vi "Read Pots.vi"() -> (2 "Right Pot":dbl, 3 "Left Pot":dbl, 4 "Right Unzeroed":dbl, 6 "Left Unzeroed":dbl)   [LabVIEW 2014]
uses:
  Robot Global Data.vi
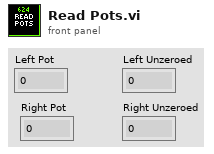
[diagram p1: front panel]
types:
  T1 = typedef "Dashboard Control Data.ctl" = cluster{"Cam Exposure":dbl, "Go to angle":dbl, "Steer PID Gains":cluster{"proportional gain (Kc)":dbl, "integral time (Ti, min)":dbl, "derivative time (Td, min)":dbl}, "Steer PID output Range":cluster{"output high":dbl, "output low":dbl}, "Pressure m \nValue":dbl, "Pressure b \nValue":dbl, "Strafe Timer\nWait":dbl, "Roller Command Cluster ":T2, "Elevator":T3, "Strafe Correct min X":dbl, "IMU Enable":bool, "Encoder Control":T5}
  T2 = typedef "Roller Control.ctl" = cluster{"Left Roller Speed":dbl, "Right Roller Speed":dbl, "Left Roller Speed Back":dbl, "Right Roller Speed Back":dbl, "Roller Align Decide Limit":u32, "Left Roller Speed Unload":dbl, "Right Roller Speed Unload":dbl, "Ping Dist Difference":dbl, "Ping In Dist":dbl, "Right Pot 0":dbl, "Pot Threshold":dbl, "Left Pot 0":dbl, "Manual 0s?":bool, "Right Pot Scale":dbl, "Left Pot Scale":dbl, "0 wait time":i32, "Reset?":bool}
  T3 = typedef "Elevator DB Control.ctl" = cluster{"PID Output Range":cluster{"output high":dbl, "output low":dbl}, "PID gains":cluster{"proportional gain (Kc)":dbl, "integral time (Ti, min)":dbl, "derivative time (Td, min)":dbl}, "Height Tolerance":dbl, " Encoder Constant":dbl, "Safe Mode Max Speed":dbl, "Eject Time":dbl, "Encoder Filter?":bool, "Zeroing Speed":dbl, "Presets":T4}
  T4 = typedef "Elevator Presets.ctl" = cluster{"Hold Tote":dbl, "Hold Trashcan":dbl, "Pickup 2 w/ Tote":dbl, "Pickup 2 w/ Trashcan":dbl, "Pickup 3 w/ Tote":dbl, "Pickup 3 w/ Trashcan":dbl, "Bottom":dbl, "Pickup 1 w/ Tote":dbl, "Pickup Trashcan":dbl, "Pickup 1 w/ Trashcan":dbl, "Eject":dbl}
  T5 = typedef "Encoder Control.ctl" = cluster{"Left Tick Constant":dbl, "Right Tick Constant":dbl, "Center Tick Constant":dbl, "Reset?":bool}
  T6 = typedef "WPI_PotentiometerDevRef.ctl" = cluster{"DevStatus":errorcluster, "Controller":T7, "Analog Channel":T8, "Invert Output":bool}
  T7 = typedef "FPGA_TypedefAnalogModule.ctl" = enum16{"Controller 1"}
  T8 = typedef "FPGA_AIChannel.ctl" = enum8{"AI 0", "AI 1", "AI 2", "AI 3", "AI MXP 0", "AI MXP 1", "AI MXP 2", "AI MXP 3", "Invalid"}
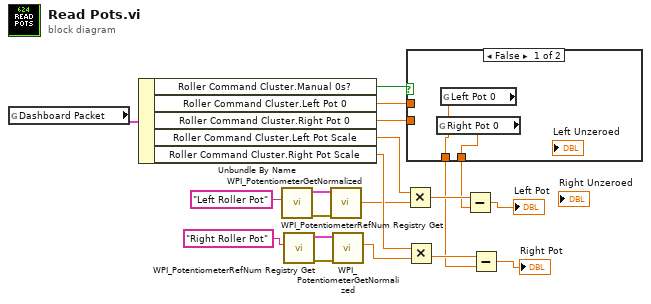
[diagram p0: block diagram]
diagram:
  n1 = global read "Robot Global Data.vi" "Dashboard Packet"() -> (w14:T1)
  n2 = Unbundle By Name(w14) -> ("Roller Command Cluster.Manual 0s?"=w5:bool, "Roller Command Cluster.Left Pot 0"=w4:dbl, "Roller Command Cluster.Right Pot 0"=w2:dbl, "Roller Command Cluster.Left Pot Scale"=w13:dbl, "Roller Command Cluster.Right Pot Scale"=w12:dbl)
  n3 = call <vilib>:"WPI_PotentiometerRefNum Registry Get.vi"("refnum name"="Left Roller Pot") -> ("error out"=w17:errorcluster, "PotDevRef"=w18:T6)  [unwired: 9 in]
  n4 = call <vilib>:"WPI_PotentiometerRefNum Registry Get.vi"("refnum name"="Right Roller Pot") -> ("error out"=w20:errorcluster, "PotDevRef"=w19:T6)  [unwired: 9 in]
  n5 = call <vilib>:"WPI_PotentiometerGetNormalized.vi"("error in"=w17, "PotDevRef"=w18) -> ("Normalized Value"=w10:dbl)  [unwired: 7 in, 2 out]
  n6 = call <vilib>:"WPI_PotentiometerGetNormalized.vi"("error in"=w20, "PotDevRef"=w19) -> ("Normalized Value"=w11:dbl)  [unwired: 7 in, 2 out]
  n7 = Multiply(x=w13, y=w10) -> (x*y=w8:dbl)
  n8 = Multiply(x=w12, y=w11) -> (x*y=w7:dbl)
  n9 = case shown="False" w5 {
    tunnel: [w21 w24] -> w3
    tunnel: w4 -> [_ w24]
    tunnel: [w22 w23] -> w1
    tunnel: w2 -> [_ w23]
    frame False {
      n10 = global read "Robot Global Data.vi" "Right Pot 0"() -> (w21:dbl)
      n11 = global read "Robot Global Data.vi" "Left Pot 0"() -> (w22:dbl)
    }
    frame True {
    }
  }
  n12 = Subtract(x=w8, y=w3) -> (x-y=→"Left Pot":dbl)
  n13 = Subtract(x=w7, y=w1) -> (x-y=→"Right Pot":dbl)
